vi "water bowl.vi"() -> ()   [LabVIEW 2018]
uses:
  <vilib>/MakerHub/LINX/Public/Peripherals/Analog/Analog Read 1 Chan.vi
  <vilib>/MakerHub/LINX/Public/Peripherals/Digital/Digital Write 1 Chan.vi
  <vilib>/MakerHub/LINX/Public/Peripherals/Analog/Analog Read N Chans.vi
  <vilib>/MakerHub/LINX/Public/Peripherals/Digital/Digital Write N Chans.vi
  <vilib>/MakerHub/LINX/Private/Local IO/LinxAnalogRead.vi
  <vilib>/MakerHub/LINX/Public/Utilities/Check Channel.vi
  <vilib>/MakerHub/LINX/Private/Local IO/LinxDigitalWrite.vi
  <vilib>/MakerHub/LINX/Public/Utilities/Open Serial.vi
  <vilib>/MakerHub/LINX/Private/Utilties/Generate Error.vi
  <vilib>/MakerHub/LINX/LMH-LINX.lvlib
panel:
  out "Not Enough":bool
  out "Water Level":dbl(slide) scale=0.0..4.0
  in  "?":bool
  in  "Serial Port":refnum<visa-resource-name>="N/A"
  # "Water Bowl Showing Water Level"
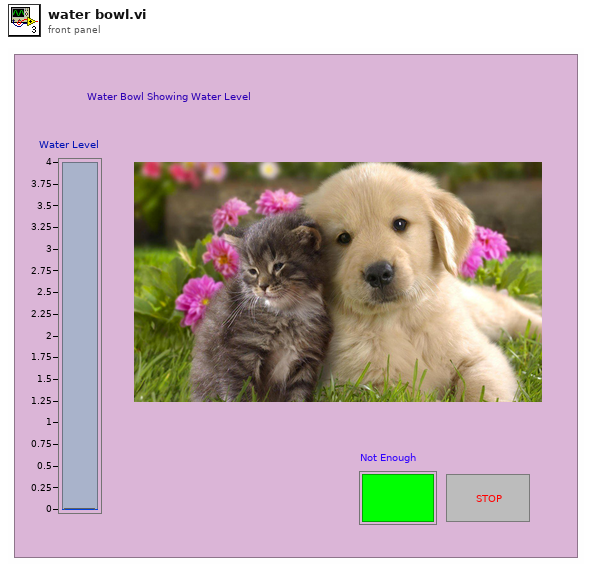
[diagram p1: front panel]
types:
  T1 = typedef "LMH-LINX.lvlib/LINX Ref.ctl" = cluster{"IO":T2, "Interface":T3, "LINX Device Config":T4}
  T2 = typedef "LMH-LINX.lvlib/Platform.ctl" = enum16{"Remote", "Local"}
  T3 = typedef "LMH-LINX.lvlib/Interface.ctl" = enum16{"Serial", "TCP"}
  T4 = typedef "LMH-LINX.lvlib/Device.lvlib/LINX Device Config.ctl" = cluster{"Interface":T3, "COM Port":refnum<visa-resource-name>, "TCP Configuration":T5, "Device Family":u8, "Device ID":u8, "Device Name":string, "TCP Ref":refnum<k5>, "Channels":T6}
  T5 = typedef "LMH-LINX.lvlib/Device.lvlib/TCP Config.ctl" = cluster{"IP Address":string, "Port":u16}
  T6 = typedef "LMH-LINX.lvlib/Channels.ctl" = cluster{"DI":u8[], "DO":u8[], "AI":u8[], "AO":u8[], "PWM":u8[], "QE":u8[], "UART":u8[], "I2C 2":u8[], "SPI":u8[], "CAN":u8[], "Servo":u8[], "AI Ref (V)":dbl, "AI Resolution (Bits)":u8, "AO Ref (V)":dbl, "AO Resolution (Bits)":u8}
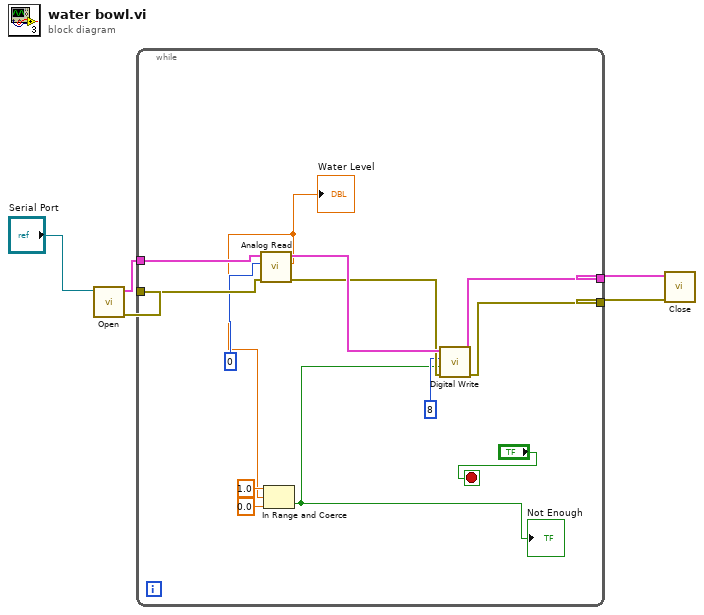
[diagram p0: block diagram]
diagram:
  n1 = call-poly <vilib>:"Open.vi"("Serial Port"="Serial Port") -> ("Error Out"=w3:errorcluster, "LINX Resource"=w5:T1)  [unwired: 8 in, 1 out]
  n2 = while {
    tunnel: w5 -> [w17]
    tunnel: [w11] -> w4
    tunnel: w3 -> [w16]
    tunnel: [w9] -> w1
    stop <- "?" stop-if-true
    n3 = call-poly <vilib>:"Analog Read.vi"("Error In"=w16, "Analog Channel"=u8 0, "LINX Resource"=w17) -> ("Error Out"=w10:errorcluster, "Voltage"=w6:dbl, "LINX Resource"=w12:T1)  [unwired: 5 in, 1 out]
    "Water Level" <- w6
    n4 = In Range and Coerce(upper limit=1.0, x=w6, lower limit=0.0) -> (In Range?=w7:bool)  [unwired: 1 out]
    "Not Enough" <- w7
    n5 = call-poly <vilib>:"Digital Write.vi"("Error In"=w10, "Output Value"=w7, "DO Channel"=u8 8, "LINX Resource"=w12) -> ("Error Out"=w9:errorcluster, "LINX Resource"=w11:T1)  [unwired: 6 in]
  }
  n6 = call <vilib>:"Close.vi"("Error In"=w1, "LINX Resource"=w4) -> ()  [unwired: 9 in, 1 out]
